vi "Gen - License Activator.vi"(8 "Error In":errorcluster, 9 "Product Name":string="VSys DAQ", 10 "License Path":path, 11 "License Param":T1) -> (0 "Error Out":errorcluster, 2 "Cancel?":bool, 3 "Updated License Param":T1)   [LabVIEW 2020]
doc: "This VI use to activate the license. User need to browse and upload a new license. The license will be validate. If valid, user able to activate."
uses:
  Control/License File Parameter.ctl
  Control/State - License Activator.ctl
  <vilib>/Utility/sysdir.llb/System Directory Type.ctl
panel:
  in  "License Status":string
  in  "Cancel":bool
  in  "Activate":bool
  in  "Upload":bool
  out "License Info":string
  in  "Done":bool
  # "ACTIVATOR"
  # "No active license"
  # "To continue this product, please update the license file provided\nby VISI and press activate. Click cancel to continue.\nVisit VISI website, www.visi.com.my to learn more."
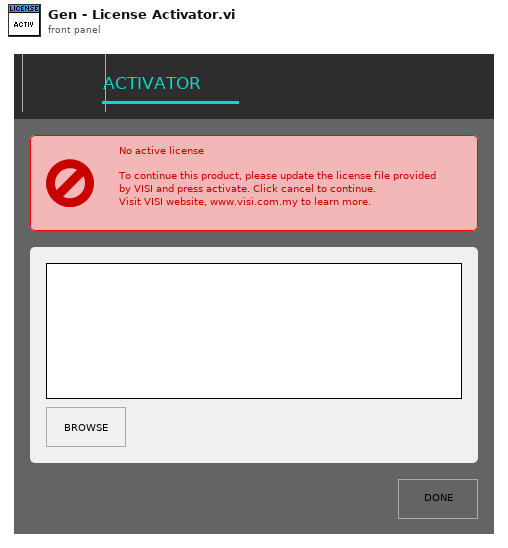
[diagram p1: front panel]
types:
  T1 = typedef "License File Parameter.ctl" = cluster{"Expired Time":string, "Computer ID":string, "Product Name":string, "Period":i16, "Activated Time":string, "License Level":enum16{"Level 1", "Level 2", "Level 3", "Level 4", "Level 5"}, "License Type":enum16{"Free", "Trial", "Subscription", "Perpetual"}, "Log Time":string}
  T2 = cluster{"T_Out":i32, "License Param (Old)":T1, "Activated?":bool, "License Param (New)":T1, "New License Path":path, "Cancel?":bool}
  T3 = typedef "State - License Activator.ctl" = enum16{"Init", "Idle", "Load New License", "Check License Info", "Activate", "Close"}
  T4 = enum8{"Enabled", "Disabled", "Disabled and Grayed Out"}
  T5 = enum16{"Level 1", "Level 2", "Level 3", "Level 4", "Level 5"}
  T6 = typedef "System Directory Type.ctl" = i32
  T7 = enum32{"invalid app kind", "Development System", "Run Time System", "Student Edition", "Embedded LabVIEW", "Evaluation", "Custom"}
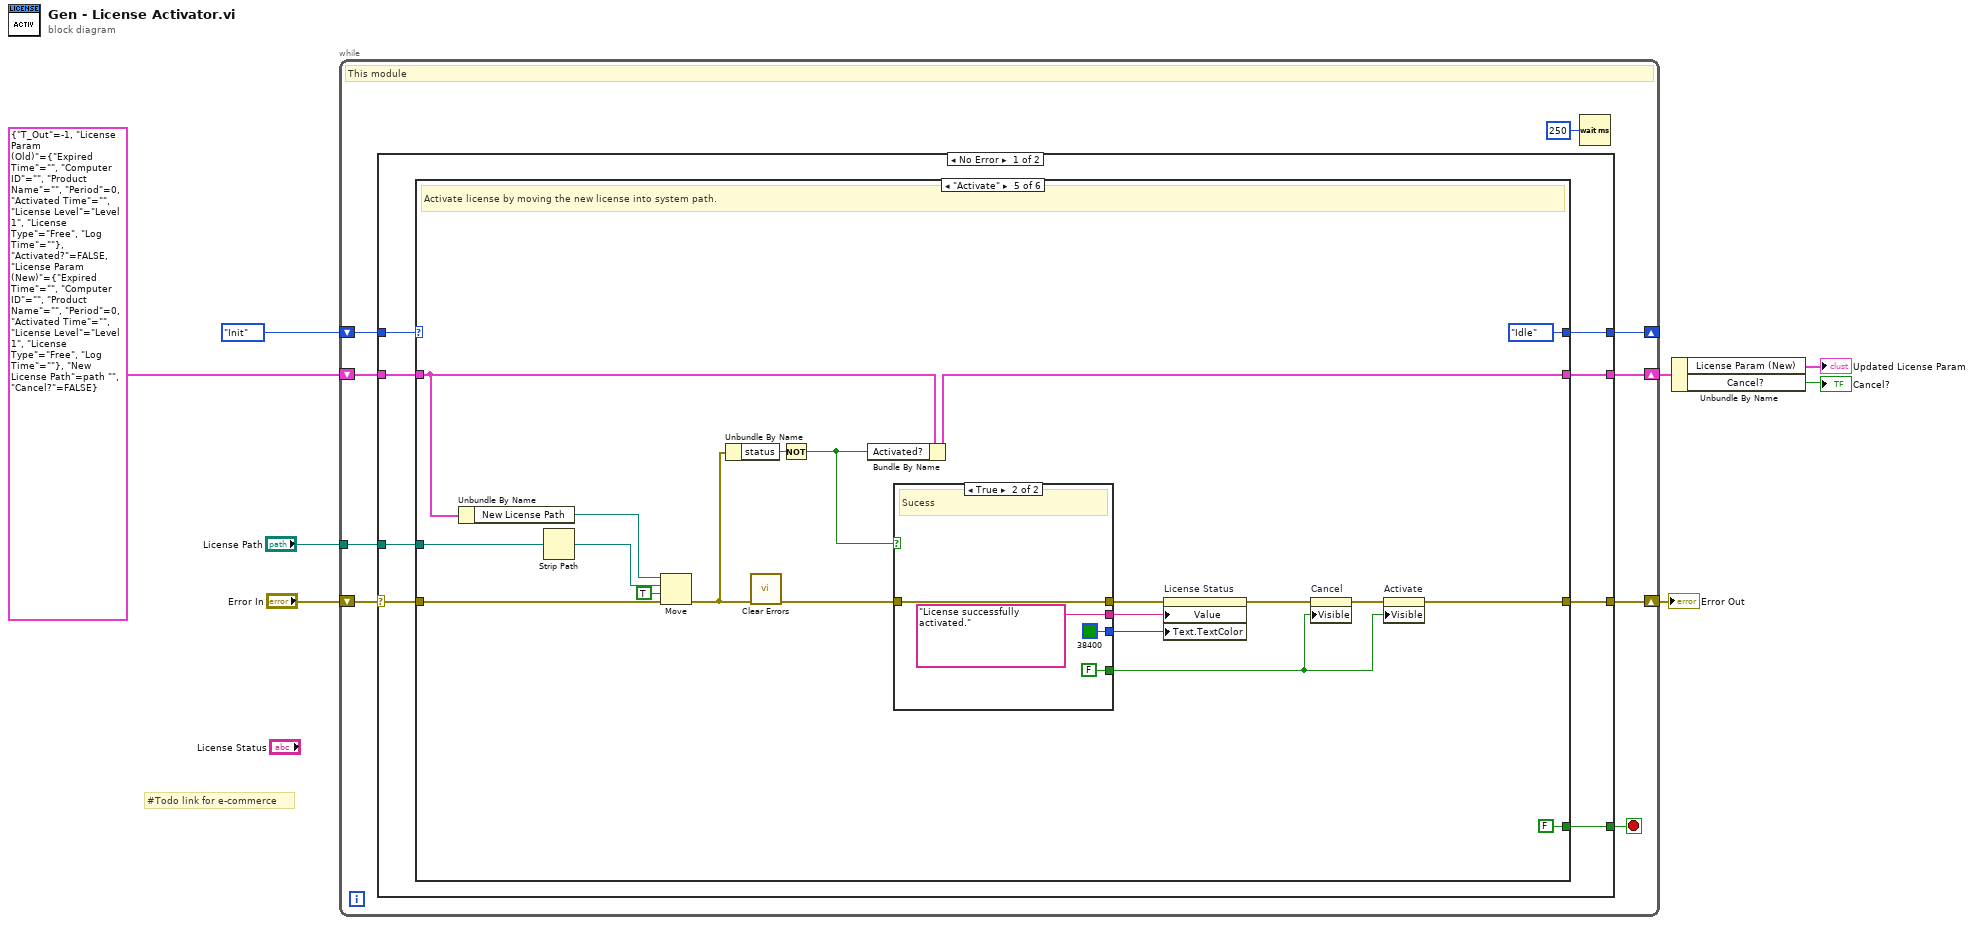
[diagram p0: block diagram]
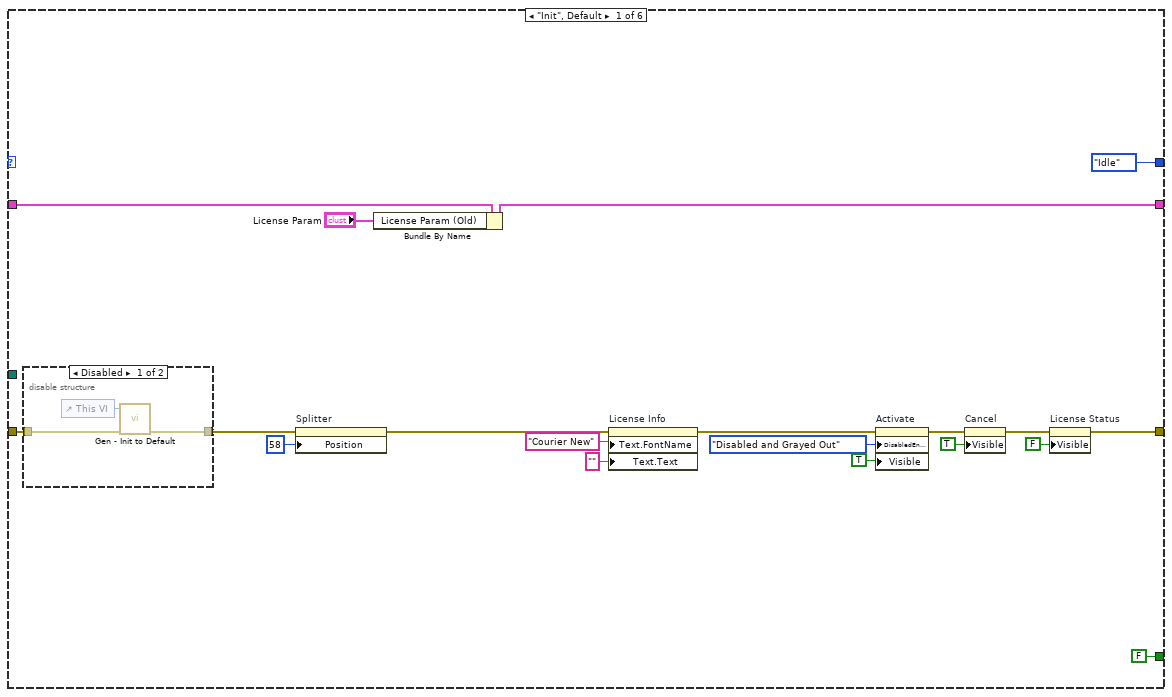
[diagram p2: hidden frame]
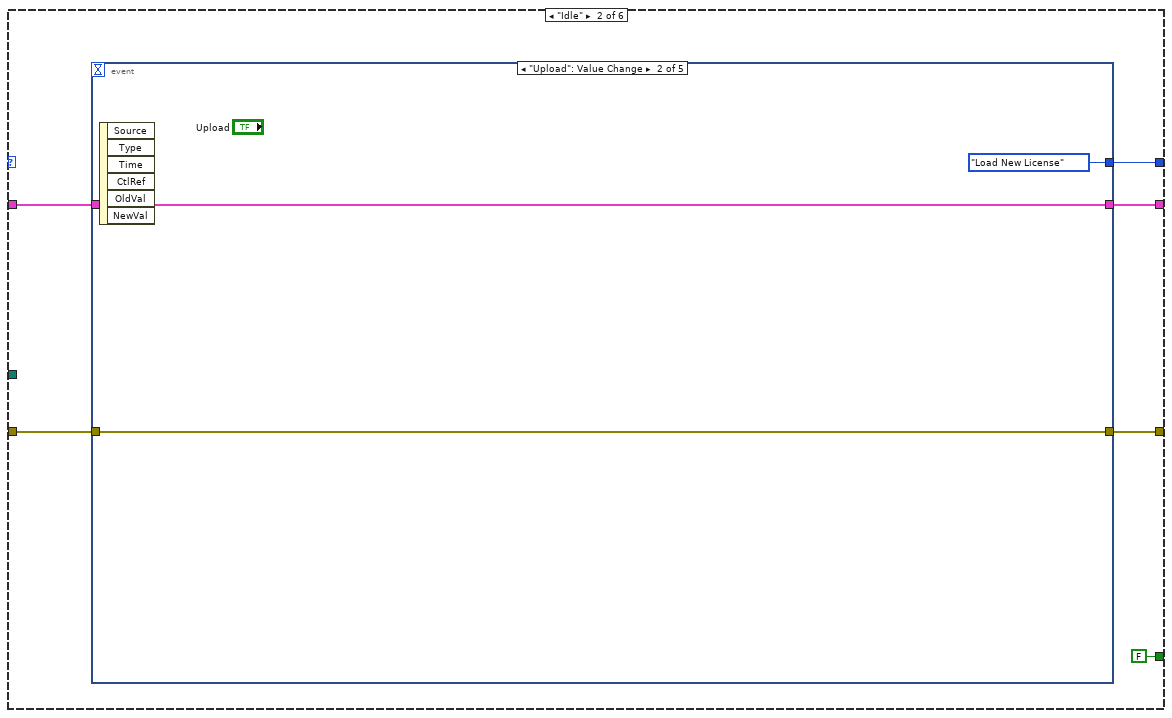
[diagram p4: hidden frame]
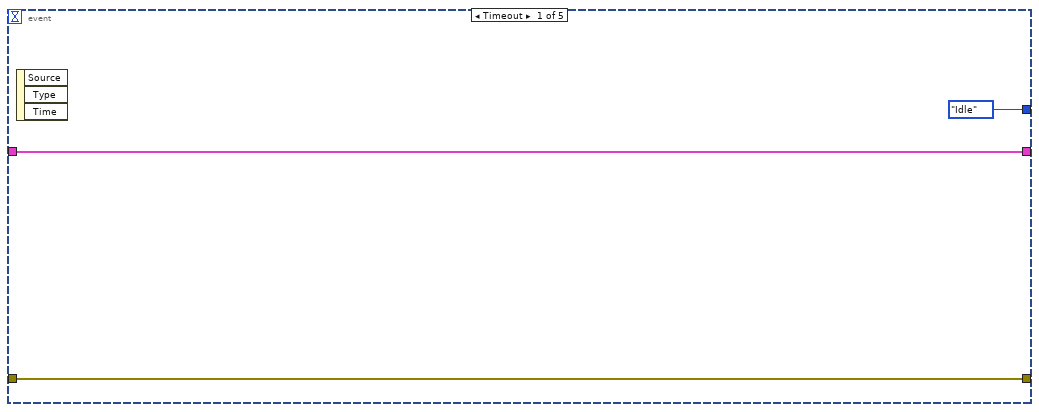
[diagram p5: hidden frame]
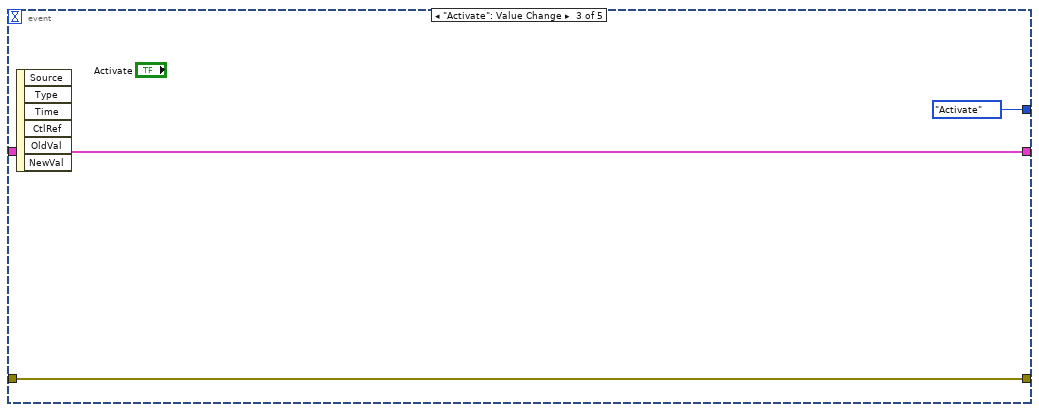
[diagram p6: hidden frame]
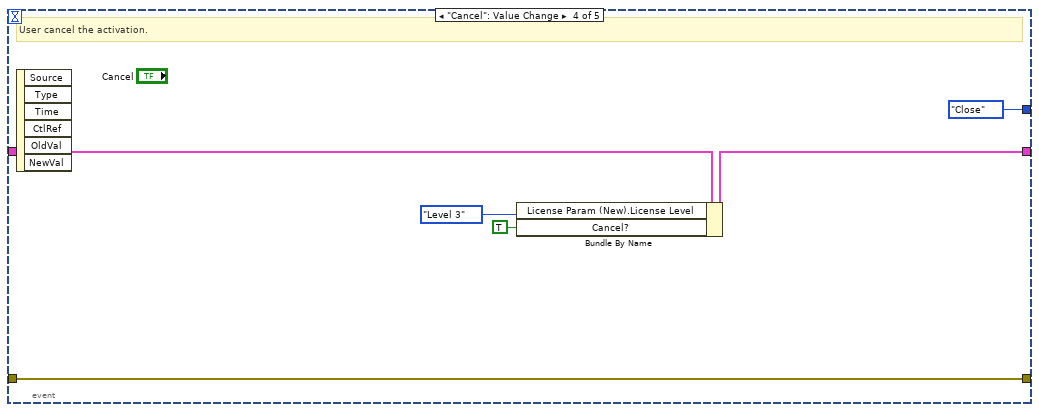
[diagram p7: hidden frame]
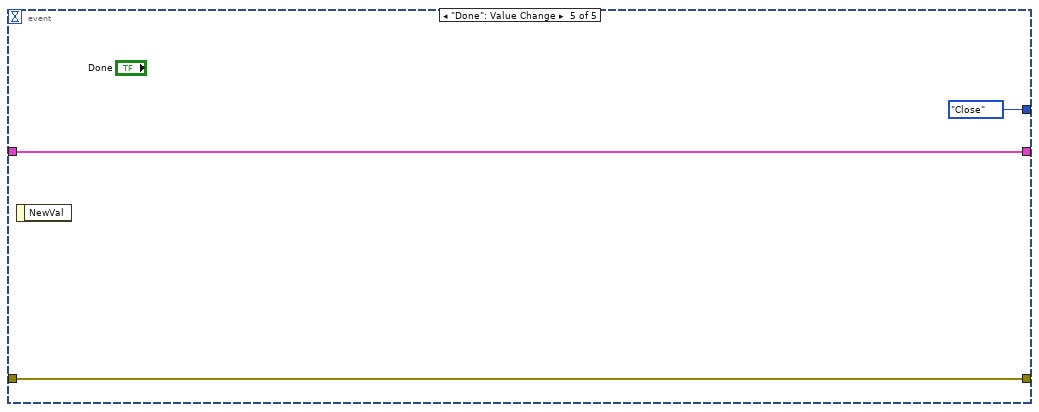
[diagram p8: hidden frame]
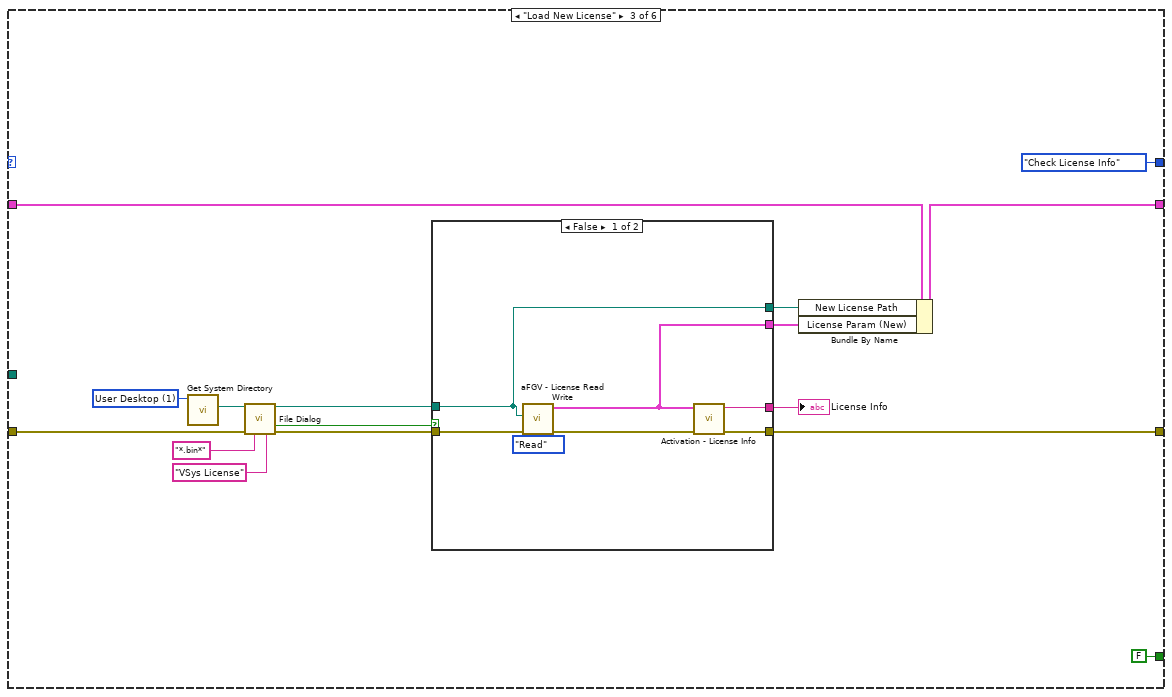
[diagram p9: hidden frame]
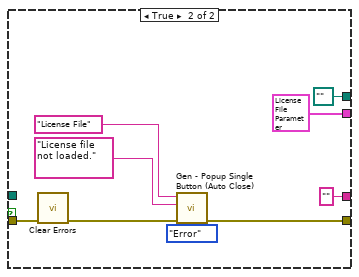
[diagram p10: hidden frame]
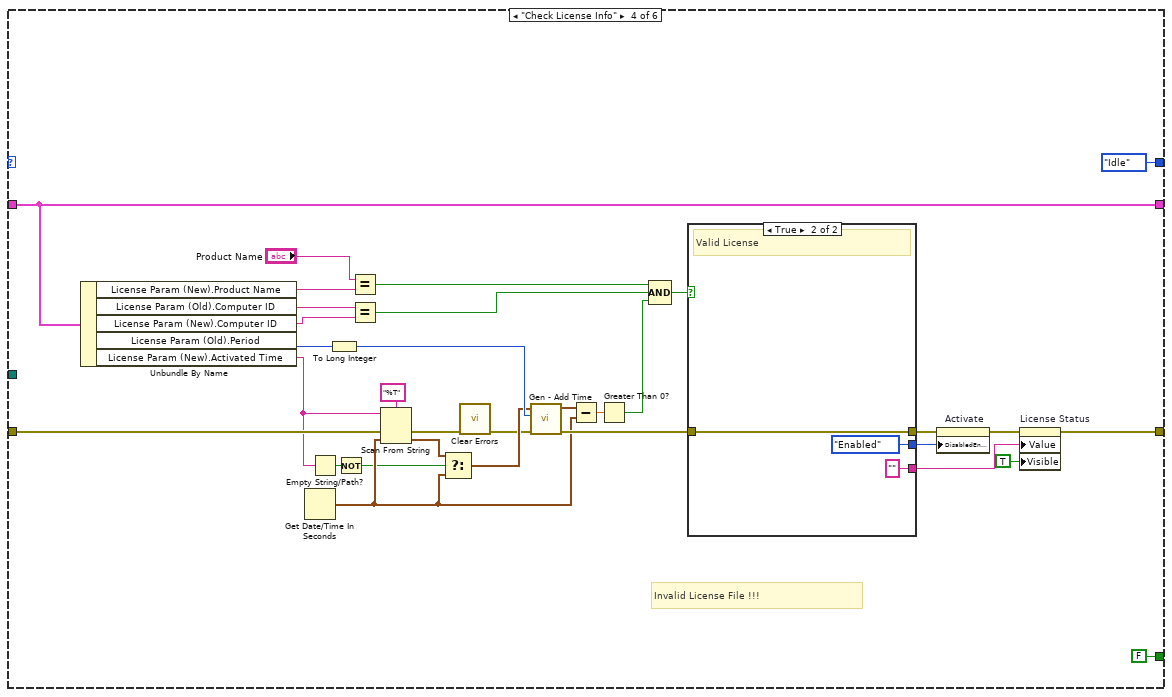
[diagram p11: hidden frame]
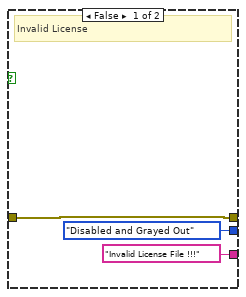
[diagram p12: hidden frame]
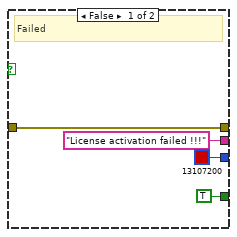
[diagram p13: hidden frame]
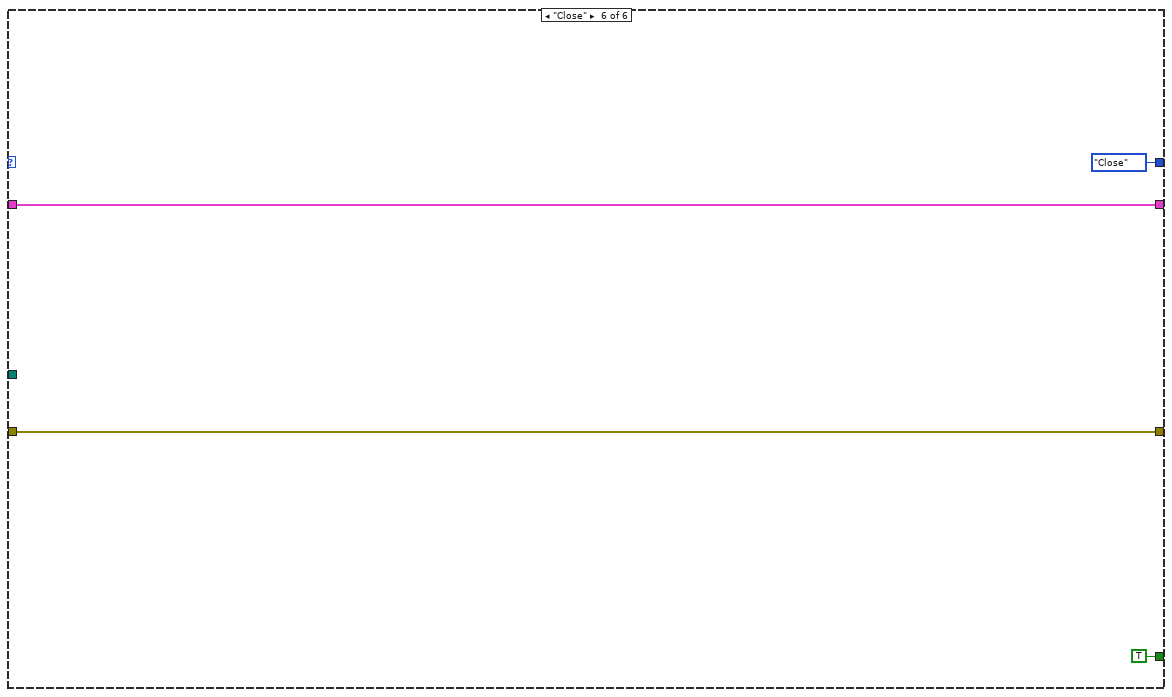
[diagram p14: hidden frame]
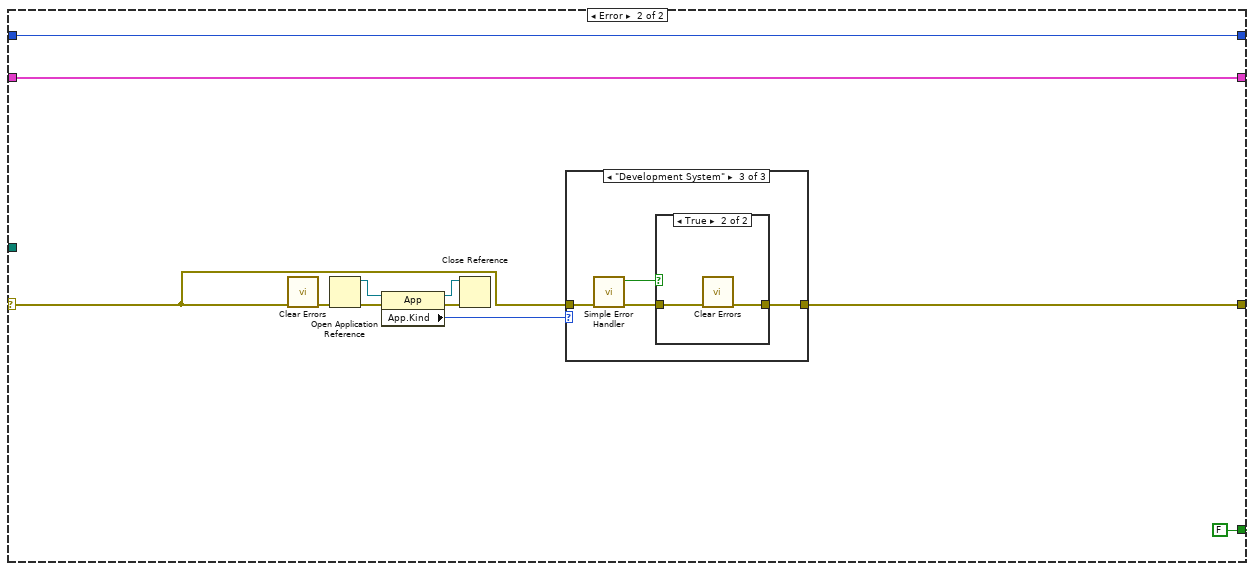
[diagram p15: hidden frame]
diagram:
  # "#Todo link for e-commerce"
  n1 = while {
    shift-right: [w13] -> _
    shift-left: State_-_License_Activator."Init" -> [w15]
    shift-right: [w16] -> w7
    shift-left: "Error In" -> [w17]
    shift-right: [w11] -> w3
    shift-left: T2 {"T_Out"=-1, "License Param (Old)"={"Expired Time"="", "Computer ID"="", "Product Name"="", "Period"=0, "Activated Time"="", "License Level"=enum."Level 1", "License Type"=enum."Free", "Log Time"=""}, "Activated?"=FALSE, "License Param (New)"={"Expired Time"="", "Computer ID"="", "Product Name"="", "Period"=0, "Activated Time"="", "License Level"=enum."Level 1", "License Type"=enum."Free", "Log Time"=""}, "New License Path"=path "", "Cancel?"=FALSE} -> [w12]
    tunnel: "License Path" -> [w9]
    stop <- w14 stop-if-true
    # "This module"
    n2 = case shown="No Error" w17 {
      selector: w17 -> [w24 w176]
      tunnel: w15 -> [w23 w184]
      tunnel: [w25 w175] -> w16
      tunnel: [w22 FALSE] -> w14
      tunnel: [w21 w184] -> w13
      tunnel: w12 -> [w20 w183]
      tunnel: [w19 w183] -> w11
      tunnel: w9 -> [w18 _]
      frame No Error {
        n3 = case shown="\"Activate\"" w23 {
          tunnel: [w31 w51 w78 w124 w148 w174] -> w25
          tunnel: w24 -> [w44 w50 w83 w118 w158 w174]
          tunnel: [FALSE FALSE FALSE FALSE FALSE TRUE] -> w22
          tunnel: [State_-_License_Activator."Idle" w54 State_-_License_Activator."Check License Info" State_-_License_Activator."Idle" State_-_License_Activator."Idle" State_-_License_Activator."Close"] -> w21
          tunnel: w20 -> [w43 w52 w88 w134 w160 w173]
          tunnel: [w34 w53 w81 w134 w154 w173] -> w19
          tunnel: w18 -> [_ _ _ _ w157 _]
          frame "Init", Default {
            n4 = disable-structure shown="Disabled" {
              disable-tunnel: w44 -> [w47 w48]
              disable-tunnel: [w45 w48] -> w28
              frame Disabled {
                n5 = control-ref of="This VI"() -> (w46:refnum<vi>)
                n6 = call "Gen - Init to Default.vi"("Error in"=w47, "This VI"=w46) -> ("Error out"=w45:errorcluster)  [unwired: 8 in, 1 out]
              }
              frame Enabled {
              }
            }
            n7 = property on="Splitter" class="Splitter"(error in=w28, "Position"=58 ("Splitter Position")) -> (error out=w27:errorcluster)  [unwired: 1 in, 1 out]
            n8 = Bundle By Name(cluster=w43, "License Param (Old)"="License Param") -> (w34:T2)
            n9 = property on="License Info" class="Str"(error in=w27, "Text.FontName"="Courier New" ("Text.Font:Name"), "Text.Text"="") -> (error out=w39:errorcluster)  [unwired: 1 in, 1 out]
            n10 = property on="Activate" class="Bool"(error in=w39, "DisabledEnum"=T4."Disabled and Grayed Out" ("Disabled"), "Visible"=TRUE) -> (error out=w37:errorcluster)  [unwired: 1 in, 1 out]
            n11 = property on="Cancel" class="Bool"(error in=w37, "Visible"=TRUE) -> (error out=w32:errorcluster)  [unwired: 1 in, 1 out]
            n12 = property on="License Status" class="Str"(error in=w32, "Visible"=FALSE) -> (error out=w31:errorcluster)  [unwired: 1 in, 1 out]
          }
          frame "Idle" {
            n13 = event shown="[1] \"Upload\": Value Change" {
              selector: _ -> [_ _ _ _ _]
              dyn-events: _ -> [_ _ _ _ _]
              timeout: _ -> [_ _ _ _ _]
              tunnel: [State_-_License_Activator."Idle" State_-_License_Activator."Load New License" State_-_License_Activator."Activate" State_-_License_Activator."Close" State_-_License_Activator."Close"] -> w54
              tunnel: [w56 w59 w62 w67 w71] -> w53
              tunnel: w52 -> [w56 w59 w62 w66 w71]
              tunnel: [w55 w58 w61 w68 w70] -> w51
              tunnel: w50 -> [w55 w58 w61 w68 w70]
              event Timeout {
                n14 = event-data() -> ()  [unwired: 1 in, 3 out]
              }
              event "Upload": Value Change {
                n15 = event-data() -> ()  [unwired: 1 in, 6 out]
              }
              event "Activate": Value Change {
                n16 = event-data() -> ()  [unwired: 1 in, 6 out]
              }
              event "Cancel": Value Change {
                # "User cancel the activation."
                n17 = event-data() -> ()  [unwired: 1 in, 6 out]
                n18 = Bundle By Name(cluster=w66, "License Param (New).License Level"=T5."Level 3", "Cancel?"=TRUE) -> (w67:T2)
              }
              event "Done": Value Change {
                n19 = event-data() -> ()  [unwired: 1 in, 1 out]
              }
            }
          }
          frame "Load New License" {
            w74 = T6 1 items=["User Home"=0, "User Desktop"=1, "User Documents"=2, "User Application Data"=3, "User Preferences"=4, "User Temporary"=5, "Public Documents"=6, "Public Application Data"=7, "Public Preferences"=8, "Public Cache"=13, "System Core Libraries"=9, "System Installed Libraries"=10, "Application Files"=11, "Boot Volume Root"=12] ("system directory type")
            n20 = call <vilib>:"Get System Directory.vi"("system directory type"=w74) -> ("system directory"=w73:path)  [unwired: 10 in]
            n21 = call "File Dialog"("start path"=w73, "error in"=w83, "pattern (all files)"="*.bin*", "pattern label"="VSys License") -> ("selected path"=w80:path, "cancelled"=w82:bool, "error out"=w84:errorcluster)  [unwired: 8 in, 1 out]
            n22 = case shown="False" w82 {
              tunnel: [w92 w101] -> w78
              tunnel: w84 -> [w94 w104]
              tunnel: [w91 T1 {"Expired Time"="", "Computer ID"="", "Product Name"="", "Period"=0, "Activated Time"="", "License Level"=enum."Level 1", "License Type"=enum."Free", "Log Time"=""} ("Data Out")] -> w79
              tunnel: w80 -> [w89 _]
              tunnel: [w90 "" ("License Info")] -> w77
              tunnel: [w89 path "" ("selected path")] -> w75
              frame False {
                n23 = call "aFGV - License Read Write.vi"("State"=enum16{"Read", "Write"}."Read", "Error In"=w94, "Path"=w89) -> ("Error Out"=w93:errorcluster, "Data Out"=w91:T1)  [unwired: 7 in]
                n24 = call "Activation - License Info.vi"("Error In"=w93, "License Param"=w91) -> ("Error Out"=w92:errorcluster, "License Info"=w90:string)  [unwired: 8 in]
              }
              frame True {
                n25 = call <vilib>:"Clear Errors.vi"("error in (no error)"=w104) -> ("error out"=w102:errorcluster)  [unwired: 5 in, 1 out]
                n26 = call "Gen - Popup Single Button (Auto Close).vi"("Type"=enum16{"Error", "Info"}."Error", "Error in"=w102, "Message in"="License file not loaded.", "Header"="License File") -> ("Error out"=w101:errorcluster)  [unwired: 6 in, 1 out]
              }
            }
            "License Info" <- w77
            n27 = Bundle By Name(cluster=w88, "New License Path"=w75, "License Param (New)"=w79) -> (w81:T2)
          }
          frame "Check License Info" {
            # "Invalid License File !!!"
            n28 = Unbundle By Name(w134) -> ("License Param (New).Product Name"=w133:string, "License Param (Old).Computer ID"=w132:string, "License Param (New).Computer ID"=w131:string, "License Param (Old).Period"=w119:i16, "License Param (New).Activated Time"=w114:string)
            n29 = Get Date/Time In Seconds() -> (seconds since 1Jan1904=w112:timestamp)
            n30 = Empty String/Path?(string/path=w114) -> (empty?=w113:bool)
            n31 = To Long Integer(number=w119) -> (32bit integer=w120:i32)
            n32 = Not(x=w113) -> (.not. x?=w111:bool)
            n33 = Equal?(x="Product Name", y=w133) -> (x = y?=w130:bool)
            n34 = Equal?(x=w132, y=w131) -> (x = y?=w129:bool)
            n35 = Scan From String(format string="%T", input string=w114, error in=w118, default 1=w112) -> (error out=w121:errorcluster, output 1=w110:timestamp)  [unwired: 1 in, 2 out]
            n36 = Select(t=w110, s=w111, f=w112) -> (s? t:f=w109:timestamp)
            n37 = call <vilib>:"Clear Errors.vi"("error in (no error)"=w121) -> ("error out"=w108:errorcluster)  [unwired: 5 in, 1 out]
            n38 = call "Gen - Add Time.vi"("Error In"=w108, "#days"=w120, "Time In"=w109) -> ("Error Out"=w117:errorcluster, "Time Out"=w122:timestamp)  [unwired: 7 in]
            n39 = Subtract(x=w122, y=w112) -> (x-y=w116:dbl)
            n40 = Greater Than 0?(x=w116) -> (x > 0?=w115:bool)
            n41 = Compound Arithmetic op=AND(w130, w129, w115) -> (w128:bool)
            n42 = case shown="True" w128 {
              tunnel: [w139 w142] -> w127
              tunnel: w117 -> [w139 w142]
              tunnel: [T4."Disabled and Grayed Out" ("Disabled") T4."Enabled" ("Disabled")] -> w126
              tunnel: ["Invalid License File !!!" ""] -> w107
              frame False {
                # "Invalid License"
              }
              frame True {
                # "Valid License"
              }
            }
            n43 = property on="Activate" class="Bool"(error in=w127, "DisabledEnum"=w126) -> (error out=w125:errorcluster)  [unwired: 1 in, 1 out]
            n44 = property on="License Status" class="Str"(error in=w125, "Value"=w107, "Visible"=TRUE) -> (error out=w124:errorcluster)  [unwired: 1 in, 1 out]
          }
          frame "Activate" {
            # "Activate license by moving the new license into system path."
            n45 = Unbundle By Name(w160) -> ("New License Path"=w159:path)
            n46 = Strip Path(path=w157) -> (stripped path=w156:path)  [unwired: 1 out]
            n47 = Move(source path=w159, error in=w158, 9:TRUE ("overwrite (F)"), 10:w156) -> (error out=w155:errorcluster)  [unwired: 1 in, 2 out]
            n48 = Unbundle By Name(w155) -> ("status"=w153:bool)
            n49 = call <vilib>:"Clear Errors.vi"("error in (no error)"=w155) -> ("error out"=w149:errorcluster)  [unwired: 5 in, 1 out]
            n50 = Not(x=w153) -> (.not. x?=w150:bool)
            n51 = Bundle By Name(cluster=w160, "Activated?"=w150) -> (w154:T2)
            n52 = case shown="True" w150 {
              tunnel: [w166 w170] -> w147
              tunnel: w149 -> [w166 w170]
              tunnel: [TRUE FALSE] -> w151
              tunnel: ["License activation failed !!!" ("Header") "License successfully activated." ("Header")] -> w145
              tunnel: [u32 13107200 u32 38400] -> w143
              frame False {
                # "Failed"
              }
              frame True {
                # "Sucess"
              }
            }
            n53 = property on="License Status" class="Str"(error in=w147, "Value"=w145, "Text.TextColor"=w143) -> (error out=w146:errorcluster)  [unwired: 1 in, 1 out]
            n54 = property on="Cancel" class="Bool"(error in=w146, "Visible"=w151) -> (error out=w152:errorcluster)  [unwired: 1 in, 1 out]
            n55 = property on="Activate" class="Bool"(error in=w152, "Visible"=w151) -> (error out=w148:errorcluster)  [unwired: 1 in, 1 out]
          }
          frame "Close" {
          }
        }
      }
      frame Error {
        n56 = call <vilib>:"Clear Errors.vi"("error in (no error)"=w176) -> ("error out"=w180:errorcluster)  [unwired: 5 in, 1 out]
        n57 = Open Application Reference(8:w180) -> (0:w182:errorcluster, 3:w179:refnum<vi>)  [unwired: 3 in]
        n58 = property class="App"(reference=w179, error in=w182) -> (reference out=w178:refnum<vi>, error out=w181:errorcluster, "App.Kind"=w177:T7)
        n59 = Close Reference(reference=w178, error in (no error)=w181) -> ()  [unwired: 1 out]
        n60 = case shown="\"Development System\"" w177 {
          tunnel: [w186 w187 w191] -> w175
          tunnel: w176 -> [w186 w187 w189]
          frame "invalid app kind", Default {
          }
          frame "Run Time System" {
          }
          frame "Development System" {
            n61 = call <vilib>:"Simple Error Handler.vi"("error in (no error)"=w189) -> ("error?"=w188:bool, "error out"=w190:errorcluster)  [unwired: 4 in, 3 out]
            n62 = case shown="True" w188 {
              tunnel: [w192 w194] -> w191
              tunnel: w190 -> [w192 w193]
              frame False {
              }
              frame True {
                n63 = call <vilib>:"Clear Errors.vi"("error in (no error)"=w193) -> ("error out"=w194:errorcluster)  [unwired: 5 in, 1 out]
              }
            }
          }
        }
      }
    }
    n64 = Wait (ms)(milliseconds to wait=u32 250) -> ()  [unwired: 1 out]
  }
  "Error Out" <- w7
  n65 = Unbundle By Name(w3) -> ("License Param (New)"=→"Updated License Param":T1, "Cancel?"=→"Cancel?":bool)
